vi "FipsAdjacent.vi"() -> (11 "Fips":i32[](array[numeric]))   [LabVIEW 2017]
panel:
  out "Adjaceny":cluster{"Fips":i32, "FipsAdj":i32[]}[](array[cluster])
  out "FipsAdj":i32[](array[numeric])
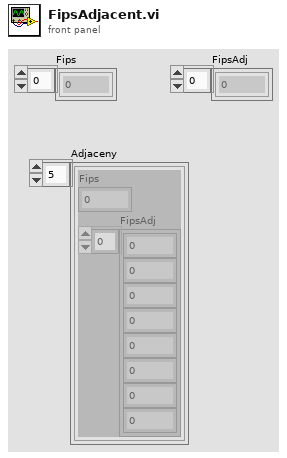
[diagram p1: front panel]
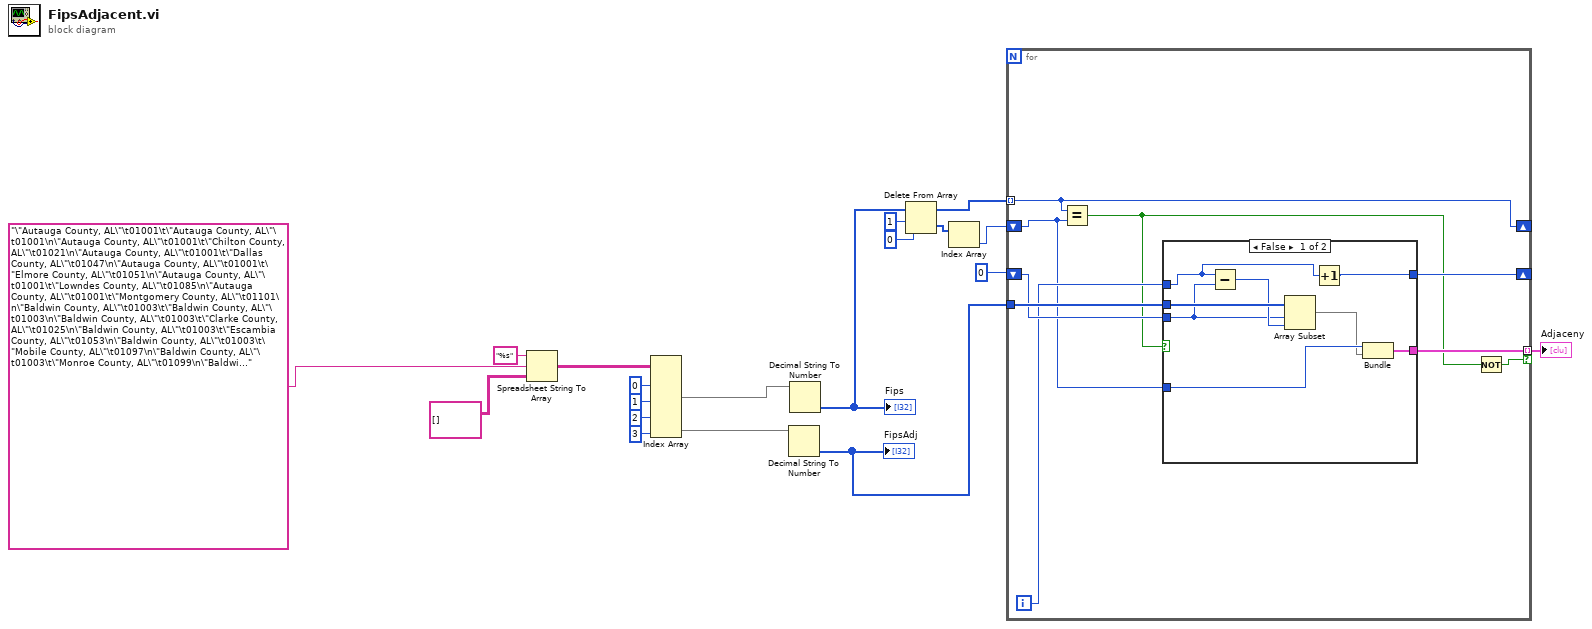
[diagram p0: block diagram]
diagram:
  n1 = Spreadsheet String To Array(format string="%s", spreadsheet string="\"Autauga County, AL\"\t01001\t\"Autauga County, AL\"\t01001\n\"Autauga County, AL\"\t01001\t\"Chilton County, AL\"\t01021\n\"Autauga County, AL\"\t01001\t\"Dallas County, AL\"\t01047\n\"Autauga County, AL\"\t01001\t\"Elmore County, AL\"\t01051\n\"Autauga County, AL\"\t01001\t\"Lowndes County, AL\"\t01085\n\"Autauga County, AL\"\t01001\t\"Montgomery County, AL\"\t01101\n\"Baldwin County, AL\"\t01003\t\"Baldwin County, AL\"\t01003\n\"Baldwin County, AL\"\t01003\t\"Clarke County, AL\"\t01025\n\"Baldwin County, AL\"\t01003\t\"Escambia County, AL\"\t01053\n\"Baldwin County, AL\"\t01003\t\"Mobile County, AL\"\t01097\n\"Baldwin County, AL\"\t01003\t\"Monroe County, AL\"\t01099\n\"Baldwin County, AL\"\t01003\t\"Washington County, AL\"\t01129\n\"Baldwin County, AL\"\t01003\t\"Escambia County, FL\"\t12033\n\"Barbour County, AL\"\t01005\t\"Barbour County, AL\"\t01005\n\"Barbour County, AL\"\t01005\t\"Bullock County, AL\"\t01011\n\"Barbour County, AL\"\t01005\t\"Dale County, AL\"\t01045\n\"Barbour County, AL\"\t01005\t\"Henry County, AL\"\t01067\n\"Barbour County, AL\"\t01005\t\"Pike County, AL\"\t01109\n\"Barbour County, AL\"\t01005\t\"Russell County, AL\"\t01113\n\"Barbour County, AL\"\t01005\t\"Clay County, GA\"\t13061\n\"Barbour County, AL\"\t01005\t\"Quitman County, GA\"\t13239\n\"Barbour County, AL\"\t01005\t\"Stewart County, GA\"\t13259\n\"Bibb County, AL\"\t01007\t\"Bibb County, AL\"\t01007\n\"Bibb County, AL\"\t01007\t\"Chilton County, AL\"\t01021\n\"Bibb County, AL\"\t01007\t\"Hale County, AL\"\t01065\n\"Bibb County, AL\"\t01007\t\"Jefferson County, AL\"\t01073\n\"Bibb County, AL\"\t01007\t\"Perry County, AL\"\t01105\n\"Bibb County, AL\"\t01007\t\"Shelby County, AL\"\t01117\n\"Bibb County, AL\"\t01007\t\"Tuscaloosa County, AL\"\t01125\n\"Blount County, AL\"\t01009\t\"Blount County, AL\"\t01009\n\"Blount County, AL\"\t01009\t\"Cullman County, AL\"\t01043\n\"Blount County, AL\"\t01009\t\"Etowah County, AL\"\t01055\n\"Blount County, AL\"\t01009\t\"Jefferson County, AL\"\t01073\n\"Blount County, AL\"\t01009\t\"Marshall County, AL\"\t01095\n\"Blount County, AL\"\t01009\t\"St. Clair County, AL\"\t01115\n\"Blount County, AL\"\t01009\t\"Walker County, AL\"\t01127\n\"Bullock County, AL\"\t01011\t\"Barbour County, AL\"\t01005\n\"Bullock County, AL\"\t01011\t\"Bullock County, AL\"\t01011\n\"Bullock County, AL\"\t01011\t\"Macon County, AL\"\t01087\n\"Bullock County, AL\"\t01011\t\"Montgomery County, AL\"\t01101\n\"Bullock County, AL\"\t01011\t\"Pike County, AL\"\t01109\n\"Bullock County, AL\"\t01011\t\"Russell County, AL\"\t01113\n\"Butler County, AL\"\t01013\t\"Butler County, AL\"\t01013\n\"Butler County, AL\"\t01013\t\"Conecuh County, AL\"\t01035\n\"Butler County, AL\"\t01013\t\"Covington County, AL\"\t01039\n\"Butler County, AL\"\t01013\t\"Crenshaw County, AL\"\t01041\n\"Butler County, AL\"\t01013\t\"Lowndes County, AL\"\t01085\n\"Butler County, AL\"\t01013\t\"Monroe County, AL\"\t01099\n\"Butler County, AL\"\t01013\t\"Wilcox County, AL\"\t01131\n\"Calhoun County, AL\"\t01015\t\"Calhoun County, AL\"\t01015\n\"Calhoun County, AL\"\t01015\t\"Cherokee County, AL\"\t01019\n\"Calhoun County, AL\"\t01015\t\"Cleburne County, AL\"\t01029\n\"Calhoun County, AL\"\t01015\t\"Etowah County, AL\"\t01055\n\"Calhoun County, AL\"\t01015\t\"St. Clair County, AL\"\t01115\n\"Calhoun County, AL\"\t01015\t\"Talladega County, AL\"\t01121\n\"Chambers County, AL\"\t01017\t\"Chambers County, AL\"\t01017\n\"Chambers County, AL\"\t01017\t\"Lee County, AL\"\t01081\n\"Chambers County, AL\"\t01017\t\"Randolph County, AL\"\t01111\n\"Chambers County, AL\"\t01017\t\"Tallapoosa County, AL\"\t01123\n\"Chambers County, AL\"\t01017\t\"Harris County, GA\"\t13145\n\"Chambers County, AL\"\t01017\t\"Troup County, GA\"\t13285\n\"Cherokee County, AL\"\t01019\t\"Calhoun County, AL\"\t01015\n\"Cherokee County, AL\"\t01019\t\"Cherokee County, AL\"\t01019\n\"Cherokee County, AL\"\t01019\t\"Cleburne County, AL\"\t01029\n\"Cherokee County, AL\"\t01019\t\"DeKalb County, AL\"\t01049\n\"Cherokee County, AL\"\t01019\t\"Etowah County, AL\"\t01055\n\"Cherokee County, AL\"\t01019\t\"Chattooga County, GA\"\t13055\n\"Cherokee County, AL\"\t01019\t\"Floyd County, GA\"\t13115\n\"Cherokee County, AL\"\t01019\t\"Polk County, GA\"\t13233\n\"Chilton County, AL\"\t01021\t\"Autauga County, AL\"\t01001\n\"Chilton County, AL\"\t01021\t\"Bibb County, AL\"\t01007\n\"Chilton County, AL\"\t01021\t\"Chilton County, AL\"\t01021\n\"Chilton County, AL\"\t01021\t\"Coosa County, AL\"\t01037\n\"Chilton County, AL\"\t01021\t\"Dallas County, AL\"\t01047\n\"Chilton County, AL\"\t01021\t\"Elmore County, AL\"\t01051\n\"Chilton County, AL\"\t01021\t\"Perry County, AL\"\t01105\n\"Chilton County, AL\"\t01021\t\"Shelby County, AL\"\t01117\n\"Choctaw County, AL\"\t01023\t\"Choctaw County, AL\"\t01023\n\"Choctaw County, AL\"\t01023\t\"Clarke County, AL\"\t01025\n\"Choctaw County, AL\"\t01023\t\"Marengo County, AL\"\t01091\n\"Choctaw County, AL\"\t01023\t\"Sumter County, AL\"\t01119\n\"Choctaw County, AL\"\t01023\t\"Washington County, AL\"\t01129\n\"Choctaw County, AL\"\t01023\t\"Clarke County, MS\"\t28023\n\"Choctaw County, AL\"\t01023\t\"Lauderdale County, MS\"\t28075\n\"Choctaw County, AL\"\t01023\t\"Wayne County, MS\"\t28153\n\"Clarke County, AL\"\t01025\t\"Baldwin County, AL\"\t01003\n\"Clarke County, AL\"\t01025\t\"Choctaw County, AL\"\t01023\n\"Clarke County, AL\"\t01025\t\"Clarke County, AL\"\t01025\n\"Clarke County, AL\"\t01025\t\"Marengo County, AL\"\t01091\n\"Clarke County, AL\"\t01025\t\"Monroe County, AL\"\t01099\n\"Clarke County, AL\"\t01025\t\"Washington County, AL\"\t01129\n\"Clarke County, AL\"\t01025\t\"Wilcox County, AL\"\t01131\n\"Clay County, AL\"\t01027\t\"Clay County, AL\"\t01027\n\"Clay County, AL\"\t01027\t\"Cleburne County, AL\"\t01029\n\"Clay County, AL\"\t01027\t\"Coosa County, AL\"\t01037\n\"Clay County, AL\"\t01027\t\"Randolph County, AL\"\t01111\n\"Clay County, AL\"\t01027\t\"Talladega County, AL\"\t01121\n\"Clay County, AL\"\t01027\t\"Tallapoosa County, AL\"\t01123\n\"Cleburne County, AL\"\t01029\t\"Calhoun County, AL\"\t01015\n\"Cleburne County, AL\"\t01029\t\"Cherokee County, AL\"\t01019\n\"Cleburne County, AL\"\t01029\t\"Clay County, AL\"\t01027\n\"Cleburne County, AL\"\t01029\t\"Cleburne County, AL\"\t01029\n\"Cleburne County, AL\"\t01029\t\"Randolph County, AL\"\t01111\n\"Cleburne County, AL\"\t01029\t\"Talladega County, AL\"\t01121\n\"Cleburne County, AL\"\t01029\t\"Carroll County, GA\"\t13045\n\"Cleburne County, AL\"\t01029\t\"Haralson County, GA\"\t13143\n\"Cleburne County, AL\"\t01029\t\"Polk County, GA\"\t13233\n\"Coffee County, AL\"\t01031\t\"Coffee County, AL\"\t01031\n\"Coffee County, AL\"\t01031\t\"Covington County, AL\"\t01039\n\"Coffee County, AL\"\t01031\t\"Crenshaw County, AL\"\t01041\n\"Coffee County, AL\"\t01031\t\"Dale County, AL\"\t01045\n\"Coffee County, AL\"\t01031\t\"Geneva County, AL\"\t01061\n\"Coffee County, AL\"\t01031\t\"Pike County, AL\"\t01109\n\"Colbert County, AL\"\t01033\t\"Colbert County, AL\"\t01033\n\"Colbert County, AL\"\t01033\t\"Franklin County, AL\"\t01059\n\"Colbert County, AL\"\t01033\t\"Lauderdale County, AL\"\t01077\n\"Colbert County, AL\"\t01033\t\"Lawrence County, AL\"\t01079\n\"Colbert County, AL\"\t01033\t\"Tishomingo County, MS\"\t28141\n\"Conecuh County, AL\"\t01035\t\"Butler County, AL\"\t01013\n\"Conecuh County, AL\"\t01035\t\"Conecuh County, AL\"\t01035\n\"Conecuh County, AL\"\t01035\t\"Covington County, AL\"\t01039\n\"Conecuh County, AL\"\t01035\t\"Escambia County, AL\"\t01053\n\"Conecuh County, AL\"\t01035\t\"Monroe County, AL\"\t01099\n\"Coosa County, AL\"\t01037\t\"Chilton County, AL\"\t01021\n\"Coosa County, AL\"\t01037\t\"Clay County, AL\"\t01027\n\"Coosa County, AL\"\t01037\t\"Coosa County, AL\"\t01037\n\"Coosa County, AL\"\t01037\t\"Elmore County, AL\"\t01051\n\"Coosa County, AL\"\t01037\t\"Shelby County, AL\"\t01117\n\"Coosa County, AL\"\t01037\t\"Talladega County, AL\"\t01121\n\"Coosa County, AL\"\t01037\t\"Tallapoosa County, AL\"\t01123\n\"Covington County, AL\"\t01039\t\"Butler County, AL\"\t01013\n\"Covington County, AL\"\t01039\t\"Coffee County, AL\"\t01031\n\"Covington County, AL\"\t01039\t\"Conecuh County, AL\"\t01035\n\"Covington County, AL\"\t01039\t\"Covington County, AL\"\t01039\n\"Covington County, AL\"\t01039\t\"Crenshaw County, AL\"\t01041\n\"Covington County, AL\"\t01039\t\"Escambia County, AL\"\t01053\n\"Covington County, AL\"\t01039\t\"Geneva County, AL\"\t01061\n\"Covington County, AL\"\t01039\t\"Okaloosa County, FL\"\t12091\n\"Covington County, AL\"\t01039\t\"Walton County, FL\"\t12131\n\"Crenshaw County, AL\"\t01041\t\"Butler County, AL\"\t01013\n\"Crenshaw County, AL\"\t01041\t\"Coffee County, AL\"\t01031\n\"Crenshaw County, AL\"\t01041\t\"Covington County, AL\"\t01039\n\"Crenshaw County, AL\"\t01041\t\"Crenshaw County, AL\"\t01041\n\"Crenshaw County, AL\"\t01041\t\"Lowndes County, AL\"\t01085\n\"Crenshaw County, AL\"\t01041\t\"Montgomery County, AL\"\t01101\n\"Crenshaw County, AL\"\t01041\t\"Pike County, AL\"\t01109\n\"Cullman County, AL\"\t01043\t\"Blount County, AL\"\t01009\n\"Cullman County, AL\"\t01043\t\"Cullman County, AL\"\t01043\n\"Cullman County, AL\"\t01043\t\"Lawrence County, AL\"\t01079\n\"Cullman County, AL\"\t01043\t\"Marshall County, AL\"\t01095\n\"Cullman County, AL\"\t01043\t\"Morgan County, AL\"\t01103\n\"Cullman County, AL\"\t01043\t\"Walker County, AL\"\t01127\n\"Cullman County, AL\"\t01043\t\"Winston County, AL\"\t01133\n\"Dale County, AL\"\t01045\t\"Barbour County, AL\"\t01005\n\"Dale County, AL\"\t01045\t\"Coffee County, AL\"\t01031\n\"Dale County, AL\"\t01045\t\"Dale County, AL\"\t01045\n\"Dale County, AL\"\t01045\t\"Geneva County, AL\"\t01061\n\"Dale County, AL\"\t01045\t\"Henry County, AL\"\t01067\n\"Dale County, AL\"\t01045\t\"Houston County, AL\"\t01069\n\"Dale County, AL\"\t01045\t\"Pike County, AL\"\t01109\n\"Dallas County, AL\"\t01047\t\"Autauga County, AL\"\t01001\n\"Dallas County, AL\"\t01047\t\"Chilton County, AL\"\t01021\n\"Dallas County, AL\"\t01047\t\"Dallas County, AL\"\t01047\n\"Dallas County, AL\"\t01047\t\"Lowndes County, AL\"\t01085\n\"Dallas County, AL\"\t01047\t\"Marengo County, AL\"\t01091\n\"Dallas County, AL\"\t01047\t\"Perry County, AL\"\t01105\n\"Dallas County, AL\"\t01047\t\"Wilcox County, AL\"\t01131\n\"DeKalb County, AL\"\t01049\t\"Cherokee County, AL\"\t01019\n\"DeKalb County, AL\"\t01049\t\"DeKalb County, AL\"\t01049\n\"DeKalb County, AL\"\t01049\t\"Etowah County, AL\"\t01055\n\"DeKalb County, AL\"\t01049\t\"Jackson County, AL\"\t01071\n\"DeKalb County, AL\"\t01049\t\"Marshall County, AL\"\t01095\n\"DeKalb County, AL\"\t01049\t\"Chattooga County, GA\"\t13055\n\"DeKalb County, AL\"\t01049\t\"Dade County, GA\"\t13083\n\"DeKalb County, AL\"\t01049\t\"Walker County, GA\"\t13295\n\"Elmore County, AL\"\t01051\t\"Autauga County, AL\"\t01001\n\"Elmore County, AL\"\t01051\t\"Chilton County, AL\"\t01021\n\"Elmore County, AL\"\t01051\t\"Coosa County, AL\"\t01037\n\"Elmore County, AL\"\t01051\t\"Elmore County, AL\"\t01051\n\"Elmore County, AL\"\t01051\t\"Macon County, AL\"\t01087\n\"Elmore County, AL\"\t01051\t\"Montgomery County, AL\"\t01101\n\"Elmore County, AL\"\t01051\t\"Tallapoosa County, AL\"\t01123\n\"Escambia County, AL\"\t01053\t\"Baldwin County, AL\"\t01003\n\"Escambia County, AL\"\t01053\t\"Conecuh County, AL\"\t01035\n\"Escambia County, AL\"\t01053\t\"Covington County, AL\"\t01039\n\"Escambia County, AL\"\t01053\t\"Escambia County, AL\"\t01053\n\"Escambia County, AL\"\t01053\t\"Monroe County, AL\"\t01099\n\"Escambia County, AL\"\t01053\t\"Escambia County, FL\"\t12033\n\"Escambia County, AL\"\t01053\t\"Okaloosa County, FL\"\t12091\n\"Escambia County, AL\"\t01053\t\"Santa Rosa County, FL\"\t12113\n\"Etowah County, AL\"\t01055\t\"Blount County, AL\"\t01009\n\"Etowah County, AL\"\t01055\t\"Calhoun County, AL\"\t01015\n\"Etowah County, AL\"\t01055\t\"Cherokee County, AL\"\t01019\n\"Etowah County, AL\"\t01055\t\"DeKalb County, AL\"\t01049\n\"Etowah County, AL\"\t01055\t\"Etowah County, AL\"\t01055\n\"Etowah County, AL\"\t01055\t\"Marshall County, AL\"\t01095\n\"Etowah County, AL\"\t01055\t\"St. Clair County, AL\"\t01115\n\"Fayette County, AL\"\t01057\t\"Fayette County, AL\"\t01057\n\"Fayette County, AL\"\t01057\t\"Lamar County, AL\"\t01075\n\"Fayette County, AL\"\t01057\t\"Marion County, AL\"\t01093\n\"Fayette County, AL\"\t01057\t\"Pickens County, AL\"\t01107\n\"Fayette County, AL\"\t01057\t\"Tuscaloosa County, AL\"\t01125\n\"Fayette County, AL\"\t01057\t\"Walker County, AL\"\t01127\n\"Franklin County, AL\"\t01059\t\"Colbert County, AL\"\t01033\n\"Franklin County, AL\"\t01059\t\"Franklin County, AL\"\t01059\n\"Franklin County, AL\"\t01059\t\"Lawrence County, AL\"\t01079\n\"Franklin County, AL\"\t01059\t\"Marion County, AL\"\t01093\n\"Franklin County, AL\"\t01059\t\"Winston County, AL\"\t01133\n\"Franklin County, AL\"\t01059\t\"Itawamba County, MS\"\t28057\n\"Franklin County, AL\"\t01059\t\"Tishomingo County, MS\"\t28141\n\"Geneva County, AL\"\t01061\t\"Coffee County, AL\"\t01031\n\"Geneva County, AL\"\t01061\t\"Covington County, AL\"\t01039\n\"Geneva County, AL\"\t01061\t\"Dale County, AL\"\t01045\n\"Geneva County, AL\"\t01061\t\"Geneva County, AL\"\t01061\n\"Geneva County, AL\"\t01061\t\"Houston County, AL\"\t01069\n\"Geneva County, AL\"\t01061\t\"Holmes County, FL\"\t12059\n\"Geneva County, AL\"\t01061\t\"Jackson County, FL\"\t12063\n\"Geneva County, AL\"\t01061\t\"Walton County, FL\"\t12131\n\"Greene County, AL\"\t01063\t\"Greene County, AL\"\t01063\n\"Greene County, AL\"\t01063\t\"Hale County, AL\"\t01065\n\"Greene County, AL\"\t01063\t\"Marengo County, AL\"\t01091\n\"Greene County, AL\"\t01063\t\"Pickens County, AL\"\t01107\n\"Greene County, AL\"\t01063\t\"Sumter County, AL\"\t01119\n\"Greene County, AL\"\t01063\t\"Tuscaloosa County, AL\"\t01125\n\"Hale County, AL\"\t01065\t\"Bibb County, AL\"\t01007\n\"Hale County, AL\"\t01065\t\"Greene County, AL\"\t01063\n\"Hale County, AL\"\t01065\t\"Hale County, AL\"\t01065\n\"Hale County, AL\"\t01065\t\"Marengo County, AL\"\t01091\n\"Hale County, AL\"\t01065\t\"Perry County, AL\"\t01105\n\"Hale County, AL\"\t01065\t\"Tuscaloosa County, AL\"\t01125\n\"Henry County, AL\"\t01067\t\"Barbour County, AL\"\t01005\n\"Henry County, AL\"\t01067\t\"Dale County, AL\"\t01045\n\"Henry County, AL\"\t01067\t\"Henry County, AL\"\t01067\n\"Henry County, AL\"\t01067\t\"Houston County, AL\"\t01069\n\"Henry County, AL\"\t01067\t\"Clay County, GA\"\t13061\n\"Henry County, AL\"\t01067\t\"Early County, GA\"\t13099\n\"Houston County, AL\"\t01069\t\"Dale County, AL\"\t01045\n\"Houston County, AL\"\t01069\t\"Geneva County, AL\"\t01061\n\"Houston County, AL\"\t01069\t\"Henry County, AL\"\t01067\n\"Houston County, AL\"\t01069\t\"Houston County, AL\"\t01069\n\"Houston County, AL\"\t01069\t\"Jackson County, FL\"\t12063\n\"Houston County, AL\"\t01069\t\"Early County, GA\"\t13099\n\"Houston County, AL\"\t01069\t\"Seminole County, GA\"\t13253\n\"Jackson County, AL\"\t01071\t\"DeKalb County, AL\"\t01049\n\"Jackson County, AL\"\t01071\t\"Jackson County, AL\"\t01071\n\"Jackson County, AL\"\t01071\t\"Madison County, AL\"\t01089\n\"Jackson County, AL\"\t01071\t\"Marshall County, AL\"\t01095\n\"Jackson County, AL\"\t01071\t\"Dade County, GA\"\t13083\n\"Jackson County, AL\"\t01071\t\"Franklin County, TN\"\t47051\n\"Jackson County, AL\"\t01071\t\"Marion County, TN\"\t47115\n\"Jefferson County, AL\"\t01073\t\"Bibb County, AL\"\t01007\n\"Jefferson County, AL\"\t01073\t\"Blount County, AL\"\t01009\n\"Jefferson County, AL\"\t01073\t\"Jefferson County, AL\"\t01073\n\"Jefferson County, AL\"\t01073\t\"St. Clair County, AL\"\t01115\n\"Jefferson County, AL\"\t01073\t\"Shelby County, AL\"\t01117\n\"Jefferson County, AL\"\t01073\t\"Tuscaloosa County, AL\"\t01125\n\"Jefferson County, AL\"\t01073\t\"Walker County, AL\"\t01127\n\"Lamar County, AL\"\t01075\t\"Fayette County, AL\"\t01057\n\"Lamar County, AL\"\t01075\t\"Lamar County, AL\"\t01075\n\"Lamar County, AL\"\t01075\t\"Marion County, AL\"\t01093\n\"Lamar County, AL\"\t01075\t\"Pickens County, AL\"\t01107\n\"Lamar County, AL\"\t01075\t\"Lowndes County, MS\"\t28087\n\"Lamar County, AL\"\t01075\t\"Monroe County, MS\"\t28095\n\"Lauderdale County, AL\"\t01077\t\"Colbert County, AL\"\t01033\n\"Lauderdale County, AL\"\t01077\t\"Lauderdale County, AL\"\t01077\n\"Lauderdale County, AL\"\t01077\t\"Lawrence County, AL\"\t01079\n\"Lauderdale County, AL\"\t01077\t\"Limestone County, AL\"\t01083\n\"Lauderdale County, AL\"\t01077\t\"Tishomingo County, MS\"\t28141\n\"Lauderdale County, AL\"\t01077\t\"Giles County, TN\"\t47055\n\"Lauderdale County, AL\"\t01077\t\"Hardin County, TN\"\t47071\n\"Lauderdale County, AL\"\t01077\t\"Lawrence County, TN\"\t47099\n\"Lauderdale County, AL\"\t01077\t\"Wayne County, TN\"\t47181\n\"Lawrence County, AL\"\t01079\t\"Colbert County, AL\"\t01033\n\"Lawrence County, AL\"\t01079\t\"Cullman County, AL\"\t01043\n\"Lawrence County, AL\"\t01079\t\"Franklin County, AL\"\t01059\n\"Lawrence County, AL\"\t01079\t\"Lauderdale County, AL\"\t01077\n\"Lawrence County, AL\"\t01079\t\"Lawrence County, AL\"\t01079\n\"Lawrence County, AL\"\t01079\t\"Limestone County, AL\"\t01083\n\"Lawrence County, AL\"\t01079\t\"Morgan County, AL\"\t01103\n\"Lawrence County, AL\"\t01079\t\"Winston County, AL\"\t01133\n\"Lee County, AL\"\t01081\t\"Chambers County, AL\"\t01017\n\"Lee County, AL\"\t01081\t\"Lee County, AL\"\t01081\n\"Lee County, AL\"\t01081\t\"Macon County, AL\"\t01087\n\"Lee County, AL\"\t01081\t\"Russell County, AL\"\t01113\n\"Lee County, AL\"\t01081\t\"Tallapoosa County, AL\"\t01123\n\"Lee County, AL\"\t01081\t\"Harris County, GA\"\t13145\n\"Lee County, AL\"\t01081\t\"Muscogee County, GA\"\t13215\n\"Limestone County, AL\"\t01083\t\"Lauderdale County, AL\"\t01077\n\"Limestone County, AL\"\t01083\t\"Lawrence County, AL\"\t01079\n\"Limestone County, AL\"\t01083\t\"Limestone County, AL\"\t01083\n\"Limestone County, AL\"\t01083\t\"Madison County, AL\"\t01089\n\"Limestone County, AL\"\t01083\t\"Morgan County, AL\"\t01103\n\"Limestone County, AL\"\t01083\t\"Giles County, TN\"\t47055\n\"Limestone County, AL\"\t01083\t\"Lincoln County, TN\"\t47103\n\"Lowndes County, AL\"\t01085\t\"Autauga County, AL\"\t01001\n\"Lowndes County, AL\"\t01085\t\"Butler County, AL\"\t01013\n\"Lowndes County, AL\"\t01085\t\"Crenshaw County, AL\"\t01041\n\"Lowndes County, AL\"\t01085\t\"Dallas County, AL\"\t01047\n\"Lowndes County, AL\"\t01085\t\"Lowndes County, AL\"\t01085\n\"Lowndes County, AL\"\t01085\t\"Montgomery County, AL\"\t01101\n\"Lowndes County, AL\"\t01085\t\"Wilcox County, AL\"\t01131\n\"Macon County, AL\"\t01087\t\"Bullock County, AL\"\t01011\n\"Macon County, AL\"\t01087\t\"Elmore County, AL\"\t01051\n\"Macon County, AL\"\t01087\t\"Lee County, AL\"\t01081\n\"Macon County, AL\"\t01087\t\"Macon County, AL\"\t01087\n\"Macon County, AL\"\t01087\t\"Montgomery County, AL\"\t01101\n\"Macon County, AL\"\t01087\t\"Russell County, AL\"\t01113\n\"Macon County, AL\"\t01087\t\"Tallapoosa County, AL\"\t01123\n\"Madison County, AL\"\t01089\t\"Jackson County, AL\"\t01071\n\"Madison County, AL\"\t01089\t\"Limestone County, AL\"\t01083\n\"Madison County, AL\"\t01089\t\"Madison County, AL\"\t01089\n\"Madison County, AL\"\t01089\t\"Marshall County, AL\"\t01095\n\"Madison County, AL\"\t01089\t\"Morgan County, AL\"\t01103\n\"Madison County, AL\"\t01089\t\"Franklin County, TN\"\t47051\n\"Madison County, AL\"\t01089\t\"Lincoln County, TN\"\t47103\n\"Marengo County, AL\"\t01091\t\"Choctaw County, AL\"\t01023\n\"Marengo County, AL\"\t01091\t\"Clarke County, AL\"\t01025\n\"Marengo County, AL\"\t01091\t\"Dallas County, AL\"\t01047\n\"Marengo County, AL\"\t01091\t\"Greene County, AL\"\t01063\n\"Marengo County, AL\"\t01091\t\"Hale County, AL\"\t01065\n\"Marengo County, AL\"\t01091\t\"Marengo County, AL\"\t01091\n\"Marengo County, AL\"\t01091\t\"Perry County, AL\"\t01105\n\"Marengo County, AL\"\t01091\t\"Sumter County, AL\"\t01119\n\"Marengo County, AL\"\t01091\t\"Wilcox County, AL\"\t01131\n\"Marion County, AL\"\t01093\t\"Fayette County, AL\"\t01057\n\"Marion County, AL\"\t01093\t\"Franklin County, AL\"\t01059\n\"Marion County, AL\"\t01093\t\"Lamar County, AL\"\t01075\n\"Marion County, AL\"\t01093\t\"Marion County, AL\"\t01093\n\"Marion County, AL\"\t01093\t\"Walker County, AL\"\t01127\n\"Marion County, AL\"\t01093\t\"Winston County, AL\"\t01133\n\"Marion County, AL\"\t01093\t\"Itawamba County, MS\"\t28057\n\"Marion County, AL\"\t01093\t\"Monroe County, MS\"\t28095\n\"Marshall County, AL\"\t01095\t\"Blount County, AL\"\t01009\n\"Marshall County, AL\"\t01095\t\"Cullman County, AL\"\t01043\n\"Marshall County, AL\"\t01095\t\"DeKalb County, AL\"\t01049\n\"Marshall County, AL\"\t01095\t\"Etowah County, AL\"\t01055\n\"Marshall County, AL\"\t01095\t\"Jackson County, AL\"\t01071\n\"Marshall County, AL\"\t01095\t\"Madison County, AL\"\t01089\n\"Marshall County, AL\"\t01095\t\"Marshall County, AL\"\t01095\n\"Marshall County, AL\"\t01095\t\"Morgan County, AL\"\t01103\n\"Mobile County, AL\"\t01097\t\"Baldwin County, AL\"\t01003\n\"Mobile County, AL\"\t01097\t\"Mobile County, AL\"\t01097\n\"Mobile County, AL\"\t01097\t\"Washington County, AL\"\t01129\n\"Mobile County, AL\"\t01097\t\"George County, MS\"\t28039\n\"Mobile County, AL\"\t01097\t\"Greene County, MS\"\t28041\n\"Mobile County, AL\"\t01097\t\"Jackson County, MS\"\t28059\n\"Monroe County, AL\"\t01099\t\"Baldwin County, AL\"\t01003\n\"Monroe County, AL\"\t01099\t\"Butler County, AL\"\t01013\n\"Monroe County, AL\"\t01099\t\"Clarke County, AL\"\t01025\n\"Monroe County, AL\"\t01099\t\"Conecuh County, AL\"\t01035\n\"Monroe County, AL\"\t01099\t\"Escambia County, AL\"\t01053\n\"Monroe County, AL\"\t01099\t\"Monroe County, AL\"\t01099\n\"Monroe County, AL\"\t01099\t\"Wilcox County, AL\"\t01131\n\"Montgomery County, AL\"\t01101\t\"Autauga County, AL\"\t01001\n\"Montgomery County, AL\"\t01101\t\"Bullock County, AL\"\t01011\n\"Montgomery County, AL\"\t01101\t\"Crenshaw County, AL\"\t01041\n\"Montgomery County, AL\"\t01101\t\"Elmore County, AL\"\t01051\n\"Montgomery County, AL\"\t01101\t\"Lowndes County, AL\"\t01085\n\"Montgomery County, AL\"\t01101\t\"Macon County, AL\"\t01087\n\"Montgomery County, AL\"\t01101\t\"Montgomery County, AL\"\t01101\n\"Montgomery County, AL\"\t01101\t\"Pike County, AL\"\t01109\n\"Morgan County, AL\"\t01103\t\"Cullman County, AL\"\t01043\n\"Morgan County, AL\"\t01103\t\"Lawrence County, AL\"\t01079\n\"Morgan County, AL\"\t01103\t\"Limestone County, AL\"\t01083\n\"Morgan County, AL\"\t01103\t\"Madison County, AL\"\t01089\n\"Morgan County, AL\"\t01103\t\"Marshall County, AL\"\t01095\n\"Morgan County, AL\"\t01103\t\"Morgan County, AL\"\t01103\n\"Perry County, AL\"\t01105\t\"Bibb County, AL\"\t01007\n\"Perry County, AL\"\t01105\t\"Chilton County, AL\"\t01021\n\"Perry County, AL\"\t01105\t\"Dallas County, AL\"\t01047\n\"Perry County, AL\"\t01105\t\"Hale County, AL\"\t01065\n\"Perry County, AL\"\t01105\t\"Marengo County, AL\"\t01091\n\"Perry County, AL\"\t01105\t\"Perry County, AL\"\t01105\n\"Pickens County, AL\"\t01107\t\"Fayette County, AL\"\t01057\n\"Pickens County, AL\"\t01107\t\"Greene County, AL\"\t01063\n\"Pickens County, AL\"\t01107\t\"Lamar County, AL\"\t01075\n\"Pickens County, AL\"\t01107\t\"Pickens County, AL\"\t01107\n\"Pickens County, AL\"\t01107\t\"Sumter County, AL\"\t01119\n\"Pickens County, AL\"\t01107\t\"Tuscaloosa County, AL\"\t01125\n\"Pickens County, AL\"\t01107\t\"Lowndes County, MS\"\t28087\n\"Pickens County, AL\"\t01107\t\"Noxubee County, MS\"\t28103\n\"Pike County, AL\"\t01109\t\"Barbour County, AL\"\t01005\n\"Pike County, AL\"\t01109\t\"Bullock County, AL\"\t01011\n\"Pike County, AL\"\t01109\t\"Coffee County, AL\"\t01031\n\"Pike County, AL\"\t01109\t\"Crenshaw County, AL\"\t01041\n\"Pike County, AL\"\t01109\t\"Dale County, AL\"\t01045\n\"Pike County, AL\"\t01109\t\"Montgomery County, AL\"\t01101\n\"Pike County, AL\"\t01109\t\"Pike County, AL\"\t01109\n\"Randolph County, AL\"\t01111\t\"Chambers County, AL\"\t01017\n\"Randolph County, AL\"\t01111\t\"Clay County, AL\"\t01027\n\"Randolph County, AL\"\t01111\t\"Cleburne County, AL\"\t01029\n\"Randolph County, AL\"\t01111\t\"Randolph County, AL\"\t01111\n\"Randolph County, AL\"\t01111\t\"Tallapoosa County, AL\"\t01123\n\"Randolph County, AL\"\t01111\t\"Carroll County, GA\"\t13045\n\"Randolph County, AL\"\t01111\t\"Heard County, GA\"\t13149\n\"Randolph County, AL\"\t01111\t\"Troup County, GA\"\t13285\n\"Russell County, AL\"\t01113\t\"Barbour County, AL\"\t01005\n\"Russell County, AL\"\t01113\t\"Bullock County, AL\"\t01011\n\"Russell County, AL\"\t01113\t\"Lee County, AL\"\t01081\n\"Russell County, AL\"\t01113\t\"Macon County, AL\"\t01087\n\"Russell County, AL\"\t01113\t\"Russell County, AL\"\t01113\n\"Russell County, AL\"\t01113\t\"Chattahoochee County, GA\"\t13053\n\"Russell County, AL\"\t01113\t\"Muscogee County, GA\"\t13215\n\"Russell County, AL\"\t01113\t\"Stewart County, GA\"\t13259\n\"St. Clair County, AL\"\t01115\t\"Blount County, AL\"\t01009\n\"St. Clair County, AL\"\t01115\t\"Calhoun County, AL\"\t01015\n\"St. Clair County, AL\"\t01115\t\"Etowah County, AL\"\t01055\n\"St. Clair County, AL\"\t01115\t\"Jefferson County, AL\"\t01073\n\"St. Clair County, AL\"\t01115\t\"St. Clair County, AL\"\t01115\n\"St. Clair County, AL\"\t01115\t\"Shelby County, AL\"\t01117\n\"St. Clair County, AL\"\t01115\t\"Talladega County, AL\"\t01121\n\"Shelby County, AL\"\t01117\t\"Bibb County, AL\"\t01007\n\"Shelby County, AL\"\t01117\t\"Chilton County, AL\"\t01021\n\"Shelby County, AL\"\t01117\t\"Coosa County, AL\"\t01037\n\"Shelby County, AL\"\t01117\t\"Jefferson County, AL\"\t01073\n\"Shelby County, AL\"\t01117\t\"St. Clair County, AL\"\t01115\n\"Shelby County, AL\"\t01117\t\"Shelby County, AL\"\t01117\n\"Shelby County, AL\"\t01117\t\"Talladega County, AL\"\t01121\n\"Sumter County, AL\"\t01119\t\"Choctaw County, AL\"\t01023\n\"Sumter County, AL\"\t01119\t\"Greene County, AL\"\t01063\n\"Sumter County, AL\"\t01119\t\"Marengo County, AL\"\t01091\n\"Sumter County, AL\"\t01119\t\"Pickens County, AL\"\t01107\n\"Sumter County, AL\"\t01119\t\"Sumter County, AL\"\t01119\n\"Sumter County, AL\"\t01119\t\"Kemper County, MS\"\t28069\n\"Sumter County, AL\"\t01119\t\"Lauderdale County, MS\"\t28075\n\"Sumter County, AL\"\t01119\t\"Noxubee County, MS\"\t28103\n\"Talladega County, AL\"\t01121\t\"Calhoun County, AL\"\t01015\n\"Talladega County, AL\"\t01121\t\"Clay County, AL\"\t01027\n\"Talladega County, AL\"\t01121\t\"Cleburne County, AL\"\t01029\n\"Talladega County, AL\"\t01121\t\"Coosa County, AL\"\t01037\n\"Talladega County, AL\"\t01121\t\"St. Clair County, AL\"\t01115\n\"Talladega County, AL\"\t01121\t\"Shelby County, AL\"\t01117\n\"Talladega County, AL\"\t01121\t\"Talladega County, AL\"\t01121\n\"Tallapoosa County, AL\"\t01123\t\"Chambers County, AL\"\t01017\n\"Tallapoosa County, AL\"\t01123\t\"Clay County, AL\"\t01027\n\"Tallapoosa County, AL\"\t01123\t\"Coosa County, AL\"\t01037\n\"Tallapoosa County, AL\"\t01123\t\"Elmore County, AL\"\t01051\n\"Tallapoosa County, AL\"\t01123\t\"Lee County, AL\"\t01081\n\"Tallapoosa County, AL\"\t01123\t\"Macon County, AL\"\t01087\n\"Tallapoosa County, AL\"\t01123\t\"Randolph County, AL\"\t01111\n\"Tallapoosa County, AL\"\t01123\t\"Tallapoosa County, AL\"\t01123\n\"Tuscaloosa County, AL\"\t01125\t\"Bibb County, AL\"\t01007\n\"Tuscaloosa County, AL\"\t01125\t\"Fayette County, AL\"\t01057\n\"Tuscaloosa County, AL\"\t01125\t\"Greene County, AL\"\t01063\n\"Tuscaloosa County, AL\"\t01125\t\"Hale County, AL\"\t01065\n\"Tuscaloosa County, AL\"\t01125\t\"Jefferson County, AL\"\t01073\n\"Tuscaloosa County, AL\"\t01125\t\"Pickens County, AL\"\t01107\n\"Tuscaloosa County, AL\"\t01125\t\"Tuscaloosa County, AL\"\t01125\n\"Tuscaloosa County, AL\"\t01125\t\"Walker County, AL\"\t01127\n\"Walker County, AL\"\t01127\t\"Blount County, AL\"\t01009\n\"Walker County, AL\"\t01127\t\"Cullman County, AL\"\t01043\n\"Walker County, AL\"\t01127\t\"Fayette County, AL\"\t01057\n\"Walker County, AL\"\t01127\t\"Jefferson County, AL\"\t01073\n\"Walker County, AL\"\t01127\t\"Marion County, AL\"\t01093\n\"Walker County, AL\"\t01127\t\"Tuscaloosa County, AL\"\t01125\n\"Walker County, AL\"\t01127\t\"Walker County, AL\"\t01127\n\"Walker County, AL\"\t01127\t\"Winston County, AL\"\t01133\n\"Washington County, AL\"\t01129\t\"Baldwin County, AL\"\t01003\n\"Washington County, AL\"\t01129\t\"Choctaw County, AL\"\t01023\n\"Washington County, AL\"\t01129\t\"Clarke County, AL\"\t01025\n\"Washington County, AL\"\t01129\t\"Mobile County, AL\"\t01097\n\"Washington County, AL\"\t01129\t\"Washington County, AL\"\t01129\n\"Washington County, AL\"\t01129\t\"Greene County, MS\"\t28041\n\"Washington County, AL\"\t01129\t\"Wayne County, MS\"\t28153\n\"Wilcox County, AL\"\t01131\t\"Butler County, AL\"\t01013\n\"Wilcox County, AL\"\t01131\t\"Clarke County, AL\"\t01025\n\"Wilcox County, AL\"\t01131\t\"Dallas County, AL\"\t01047\n\"Wilcox County, AL\"\t01131\t\"Lowndes County, AL\"\t01085\n\"Wilcox County, AL\"\t01131\t\"Marengo County, AL\"\t01091\n\"Wilcox County, AL\"\t01131\t\"Monroe County, AL\"\t01099\n\"Wilcox County, AL\"\t01131\t\"Wilcox County, AL\"\t01131\n\"Winston County, AL\"\t01133\t\"Cullman County, AL\"\t01043\n\"Winston County, AL\"\t01133\t\"Franklin County, AL\"\t01059\n\"Winston County, AL\"\t01133\t\"Lawrence County, AL\"\t01079\n\"Winston County, AL\"\t01133\t\"Marion County, AL\"\t01093\n\"Winston County, AL\"\t01133\t\"Walker County, AL\"\t01127\n\"Winston County, AL\"\t01133\t\"Winston County, AL\"\t01133\n\"Aleutians East Borough, AK\"\t02013\t\"Aleutians East Borough, AK\"\t02013\n\"Aleutians East Borough, AK\"\t02013\t\"Aleutians West Census Area, AK\"\t02016\n\"Aleutians East Borough, AK\"\t02013\t\"Lake and Peninsula Borough, AK\"\t02164\n\"Aleutians West Census Area, AK\"\t02016\t\"Aleutians East Borough, AK\"\t02013\n\"Aleutians West Census Area, AK\"\t02016\t\"Aleutians West Census Area, AK\"\t02016\n\"Anchorage Municipality, AK\"\t02020\t\"Anchorage Municipality, AK\"\t02020\n\"Anchorage Municipality, AK\"\t02020\t\"Kenai Peninsula Borough, AK\"\t02122\n\"Anchorage Municipality, AK\"\t02020\t\"Matanuska-Susitna Borough, AK\"\t02170\n\"Anchorage Municipality, AK\"\t02020\t\"Valdez-Cordova Census Area, AK\"\t02261\n\"Bethel Census Area, AK\"\t02050\t\"Bethel Census Area, AK\"\t02050\n\"Bethel Census Area, AK\"\t02050\t\"Dillingham Census Area, AK\"\t02070\n\"Bethel Census Area, AK\"\t02050\t\"Kenai Peninsula Borough, AK\"\t02122\n\"Bethel Census Area, AK\"\t02050\t\"Lake and Peninsula Borough, AK\"\t02164\n\"Bethel Census Area, AK\"\t02050\t\"Matanuska-Susitna Borough, AK\"\t02170\n\"Bethel Census Area, AK\"\t02050\t\"Wade Hampton Census Area, AK\"\t02270\n\"Bethel Census Area, AK\"\t02050\t\"Yukon-Koyukuk Census Area, AK\"\t02290\n\"Bristol Bay Borough, AK\"\t02060\t\"Bristol Bay Borough, AK\"\t02060\n\"Bristol Bay Borough, AK\"\t02060\t\"Dillingham Census Area, AK\"\t02070\n\"Bristol Bay Borough, AK\"\t02060\t\"Lake and Peninsula Borough, AK\"\t02164\n\"Denali Borough, AK\"\t02068\t\"Denali Borough, AK\"\t02068\n\"Denali Borough, AK\"\t02068\t\"Fairbanks North Star Borough, AK\"\t02090\n\"Denali Borough, AK\"\t02068\t\"Matanuska-Susitna Borough, AK\"\t02170\n\"Denali Borough, AK\"\t02068\t\"Southeast Fairbanks Census Area, AK\"\t02240\n\"Denali Borough, AK\"\t02068\t\"Yukon-Koyukuk Census Area, AK\"\t02290\n\"Dillingham Census Area, AK\"\t02070\t\"Bethel Census Area, AK\"\t02050\n\"Dillingham Census Area, AK\"\t02070\t\"Bristol Bay Borough, AK\"\t02060\n\"Dillingham Census Area, AK\"\t02070\t\"Dillingham Census Area, AK\"\t02070\n\"Dillingham Census Area, AK\"\t02070\t\"Lake and Peninsula Borough, AK\"\t02164\n\"Fairbanks North Star Borough, AK\"\t02090\t\"Denali Borough, AK\"\t02068\n\"Fairbanks North Star Borough, AK\"\t02090\t\"Fairbanks North Star Borough, AK\"\t02090\n\"Fairbanks North Star Borough, AK\"\t02090\t\"Southeast Fairbanks Census Area, AK\"\t02240\n\"Fairbanks North Star Borough, AK\"\t02090\t\"Yukon-Koyukuk Census Area, AK\"\t02290\n\"Haines Borough, AK\"\t02100\t\"Haines Borough, AK\"\t02100\n\"Haines Borough, AK\"\t02100\t\"Hoonah-Angoon Census Area, AK\"\t02105\n\"Haines Borough, AK\"\t02100\t\"Juneau City and Borough, AK\"\t02110\n\"Haines Borough, AK\"\t02100\t\"Skagway Municipality, AK\"\t02230\n\"Hoonah-Angoon Census Area, AK\"\t02105\t\"Haines Borough, AK\"\t02100\n\"Hoonah-Angoon Census Area, AK\"\t02105\t\"Hoonah-Angoon Census Area, AK\"\t02105\n\"Hoonah-Angoon Census Area, AK\"\t02105\t\"Juneau City and Borough, AK\"\t02110\n\"Hoonah-Angoon Census Area, AK\"\t02105\t\"Petersburg Census Area, AK\"\t02195\n\"Hoonah-Angoon Census Area, AK\"\t02105\t\"Sitka City and Borough, AK\"\t02220\n\"Hoonah-Angoon Census Area, AK\"\t02105\t\"Yakutat City and Borough, AK\"\t02282\n\"Juneau City and Borough, AK\"\t02110\t\"Haines Borough, AK\"\t02100\n\"Juneau City and Borough, AK\"\t02110\t\"Hoonah-Angoon Census Area, AK\"\t02105\n\"Juneau City and Borough, AK\"\t02110\t\"Juneau City and Borough, AK\"\t02110\n\"Kenai Peninsula Borough, AK\"\t02122\t\"Anchorage Municipality, AK\"\t02020\n\"Kenai Peninsula Borough, AK\"\t02122\t\"Bethel Census Area, AK\"\t02050\n\"Kenai Peninsula Borough, AK\"\t02122\t\"Kenai Peninsula Borough, AK\"\t02122\n\"Kenai Peninsula Borough, AK\"\t02122\t\"Kodiak Island Borough, AK\"\t02150\n\"Kenai Peninsula Borough, AK\"\t02122\t\"Lake and Peninsula Borough, AK\"\t02164\n\"Kenai Peninsula Borough, AK\"\t02122\t\"Matanuska-Susitna Borough, AK\"\t02170\n\"Kenai Peninsula Borough, AK\"\t02122\t\"Valdez-Cordova Census Area, AK\"\t02261\n\"Ketchikan Gateway Borough, AK\"\t02130\t\"Ketchikan Gateway Borough, AK\"\t02130\n\"Ketchikan Gateway Borough, AK\"\t02130\t\"Prince of Wales-Hyder Census Area, AK\"\t02198\n\"Ketchikan Gateway Borough, AK\"\t02130\t\"Wrangell City and Borough, AK\"\t02275\n\"Kodiak Island Borough, AK\"\t02150\t\"Kenai Peninsula Borough, AK\"\t02122\n\"Kodiak Island Borough, AK\"\t02150\t\"Kodiak Island Borough, AK\"\t02150\n\"Kodiak Island Borough, AK\"\t02150\t\"Lake and Peninsula Borough, AK\"\t02164\n\"Lake and Peninsula Borough, AK\"\t02164\t\"Aleutians East Borough, AK\"\t02013\n\"Lake and Peninsula Borough, AK\"\t02164\t\"Bethel Census Area, AK\"\t02050\n\"Lake and Peninsula Borough, AK\"\t02164\t\"Bristol Bay Borough, AK\"\t02060\n\"Lake and Peninsula Borough, AK\"\t02164\t\"Dillingham Census Area, AK\"\t02070\n\"Lake and Peninsula Borough, AK\"\t02164\t\"Kenai Peninsula Borough, AK\"\t02122\n\"Lake and Peninsula Borough, AK\"\t02164\t\"Kodiak Island Borough, AK\"\t02150\n\"Lake and Peninsula Borough, AK\"\t02164\t\"Lake and Peninsula Borough, AK\"\t02164\n\"Matanuska-Susitna Borough, AK\"\t02170\t\"Anchorage Municipality, AK\"\t02020\n\"Matanuska-Susitna Borough, AK\"\t02170\t\"Bethel Census Area, AK\"\t02050\n\"Matanuska-Susitna Borough, AK\"\t02170\t\"Denali Borough, AK\"\t02068\n\"Matanuska-Susitna Borough, AK\"\t02170\t\"Kenai Peninsula Borough, AK\"\t02122\n\"Matanuska-Susitna Borough, AK\"\t02170\t\"Matanuska-Susitna Borough, AK\"\t02170\n\"Matanuska-Susitna Borough, AK\"\t02170\t\"Southeast Fairbanks Census Area, AK\"\t02240\n\"Matanuska-Susitna Borough, AK\"\t02170\t\"Valdez-Cordova Census Area, AK\"\t02261\n\"Matanuska-Susitna Borough, AK\"\t02170\t\"Yukon-Koyukuk Census Area, AK\"\t02290\n\"Nome Census Area, AK\"\t02180\t\"Nome Census Area, AK\"\t02180\n\"Nome Census Area, AK\"\t02180\t\"Northwest Arctic Borough, AK\"\t02188\n\"Nome Census Area, AK\"\t02180\t\"Wade Hampton Census Area, AK\"\t02270\n\"Nome Census Area, AK\"\t02180\t\"Yukon-Koyukuk Census Area, AK\"\t02290\n\"North Slope Borough, AK\"\t02185\t\"North Slope Borough, AK\"\t02185\n\"North Slope Borough, AK\"\t02185\t\"Northwest Arctic Borough, AK\"\t02188\n\"North Slope Borough, AK\"\t02185\t\"Yukon-Koyukuk Census Area, AK\"\t02290\n\"Northwest Arctic Borough, AK\"\t02188\t\"Nome Census Area, AK\"\t02180\n\"Northwest Arctic Borough, AK\"\t02188\t\"North Slope Borough, AK\"\t02185\n\"Northwest Arctic Borough, AK\"\t02188\t\"Northwest Arctic Borough, AK\"\t02188\n\"Northwest Arctic Borough, AK\"\t02188\t\"Yukon-Koyukuk Census Area, AK\"\t02290\n\"Petersburg Census Area, AK\"\t02195\t\"Hoonah-Angoon Census Area, AK\"\t02105\n\"Petersburg Census Area, AK\"\t02195\t\"Petersburg Census Area, AK\"\t02195\n\"Petersburg Census Area, AK\"\t02195\t\"Prince of Wales-Hyder Census Area, AK\"\t02198\n\"Petersburg Census Area, AK\"\t02195\t\"Sitka City and Borough, AK\"\t02220\n\"Petersburg Census Area, AK\"\t02195\t\"Wrangell City and Borough, AK\"\t02275\n\"Prince of Wales-Hyder Census Area, AK\"\t02198\t\"Ketchikan Gateway Borough, AK\"\t02130\n\"Prince of Wales-Hyder Census Area, AK\"\t02198\t\"Petersburg Census Area, AK\"\t02195\n\"Prince of Wales-Hyder Census Area, AK\"\t02198\t\"Prince of Wales-Hyder Census Area, AK\"\t02198\n\"Prince of Wales-Hyder Census Area, AK\"\t02198\t\"Wrangell City and Borough, AK\"\t02275\n\"Sitka City and Borough, AK\"\t02220\t\"Hoonah-Angoon Census Area, AK\"\t02105\n\"Sitka City and Borough, AK\"\t02220\t\"Petersburg Census Area, AK\"\t02195\n\"Sitka City and Borough, AK\"\t02220\t\"Sitka City and Borough, AK\"\t02220\n\"Skagway Municipality, AK\"\t02230\t\"Haines Borough, AK\"\t02100\n\"Skagway Municipality, AK\"\t02230\t\"Skagway Municipality, AK\"\t02230\n\"Southeast Fairbanks Census Area, AK\"\t02240\t\"Denali Borough, AK\"\t02068\n\"Southeast Fairbanks Census Area, AK\"\t02240\t\"Fairbanks North Star Borough, AK\"\t02090\n\"Southeast Fairbanks Census Area, AK\"\t02240\t\"Matanuska-Susitna Borough, AK\"\t02170\n\"Southeast Fairbanks Census Area, AK\"\t02240\t\"Southeast Fairbanks Census Area, AK\"\t02240\n\"Southeast Fairbanks Census Area, AK\"\t02240\t\"Valdez-Cordova Census Area, AK\"\t02261\n\"Southeast Fairbanks Census Area, AK\"\t02240\t\"Yukon-Koyukuk Census Area, AK\"\t02290\n\"Valdez-Cordova Census Area, AK\"\t02261\t\"Anchorage Municipality, AK\"\t02020\n\"Valdez-Cordova Census Area, AK\"\t02261\t\"Kenai Peninsula Borough, AK\"\t02122\n\"Valdez-Cordova Census Area, AK\"\t02261\t\"Matanuska-Susitna Borough, AK\"\t02170\n\"Valdez-Cordova Census Area, AK\"\t02261\t\"Southeast Fairbanks Census Area, AK\"\t02240\n\"Valdez-Cordova Census Area, AK\"\t02261\t\"Valdez-Cordova Census Area, AK\"\t02261\n\"Valdez-Cordova Census Area, AK\"\t02261\t\"Yakutat City and Borough, AK\"\t02282\n\"Wade Hampton Census Area, AK\"\t02270\t\"Bethel Census Area, AK\"\t02050\n\"Wade Hampton Census Area, AK\"\t02270\t\"Nome Census Area, AK\"\t02180\n\"Wade Hampton Census Area, AK\"\t02270\t\"Wade Hampton Census Area, AK\"\t02270\n\"Wade Hampton Census Area, AK\"\t02270\t\"Yukon-Koyukuk Census Area, AK\"\t02290\n\"Wrangell City and Borough, AK\"\t02275\t\"Ketchikan Gateway Borough, AK\"\t02130\n\"Wrangell City and Borough, AK\"\t02275\t\"Petersburg Census Area, AK\"\t02195\n\"Wrangell City and Borough, AK\"\t02275\t\"Prince of Wales-Hyder Census Area, AK\"\t02198\n\"Wrangell City and Borough, AK\"\t02275\t\"Wrangell City and Borough, AK\"\t02275\n\"Yakutat City and Borough, AK\"\t02282\t\"Hoonah-Angoon Census Area, AK\"\t02105\n\"Yakutat City and Borough, AK\"\t02282\t\"Valdez-Cordova Census Area, AK\"\t02261\n\"Yakutat City and Borough, AK\"\t02282\t\"Yakutat City and Borough, AK\"\t02282\n\"Yukon-Koyukuk Census Area, AK\"\t02290\t\"Bethel Census Area, AK\"\t02050\n\"Yukon-Koyukuk Census Area, AK\"\t02290\t\"Denali Borough, AK\"\t02068\n\"Yukon-Koyukuk Census Area, AK\"\t02290\t\"Fairbanks North Star Borough, AK\"\t02090\n\"Yukon-Koyukuk Census Area, AK\"\t02290\t\"Matanuska-Susitna Borough, AK\"\t02170\n\"Yukon-Koyukuk Census Area, AK\"\t02290\t\"Nome Census Area, AK\"\t02180\n\"Yukon-Koyukuk Census Area, AK\"\t02290\t\"North Slope Borough, AK\"\t02185\n\"Yukon-Koyukuk Census Area, AK\"\t02290\t\"Northwest Arctic Borough, AK\"\t02188\n\"Yukon-Koyukuk Census Area, AK\"\t02290\t\"Southeast Fairbanks Census Area, AK\"\t02240\n\"Yukon-Koyukuk Census Area, AK\"\t02290\t\"Wade Hampton Census Area, AK\"\t02270\n\"Yukon-Koyukuk Census Area, AK\"\t02290
